vi "Init.vi"(0 "STOMP in":refnum<class "STOMP.lvclass">, 5 "error in (no error)":errorcluster) -> (14 "STOMP out":refnum<class "STOMP.lvclass">, 19 "error out":errorcluster)   [LabVIEW 2017, in "STOMP.lvclass"]
uses:
  STOMP.lvclass
  Typedefs/Type_ServerFrame.ctl
  Typedefs/Type_ServerFrameType.ctl
  Typedefs/ObjectAttributes.ctl
  Typedefs/Type_ActiveSubscription.ctl
  Typedefs/Type_AckHeader.ctl
  Typedefs/Type_FrameHeader.ctl
  STOMP.lvclass/STOMP.ctl
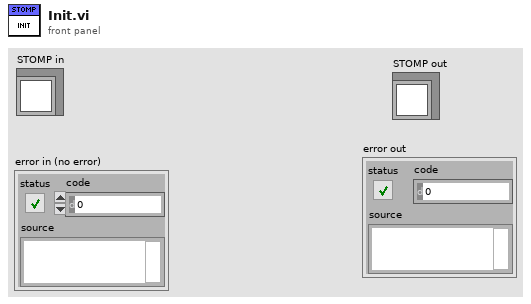
[diagram p1: front panel]
types:
  T1 = typedef "STOMP.lvclass/ObjectAttributes.ctl" = cluster{"address":string, "port":u16, "ConnectionRef":refnum<k5>, "messageQueue":refnum<queue>, "receiptQueue":refnum<queue>, "errorQueue":refnum<queue>, "sendQueue":refnum<queue>, "currentReceiptNumber":u64, "currentSubscriptionId":u64, "closeConnection":bool, "activeSubscriptions":T2[]}
  T2 = typedef "STOMP.lvclass/Type_ActiveSubscription.ctl" = cluster{"id":u64, "receipt":bool, "Destination":string, "ack":T3, "headers":T4[]}
  T3 = typedef "STOMP.lvclass/Type_AckHeader.ctl" = enum16{"auto", "client", "client-individual"}
  T4 = typedef "STOMP.lvclass/Type_FrameHeader.ctl" = cluster{"Header":string, "Value":string}
  T5 = typedef "STOMP.lvclass/Type_ServerFrame.ctl" = cluster{"Type":T6, "Headers":cluster{"Header":string, "Value":string}[], "Body":string}
  T6 = typedef "STOMP.lvclass/Type_ServerFrameType.ctl" = enum16{"Undefined", "MESSAGE", "CONNECTED", "RECEIPT", "ERROR"}
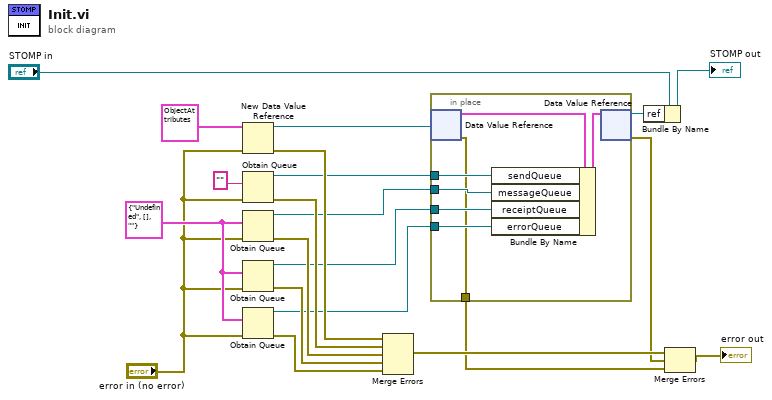
[diagram p0: block diagram]
diagram:
  w20 = T5 {"Type"=enum."Undefined", "Headers"=[], "Body"=""} ("Type_ServerFrame")
  n1 = New Data Value Reference(data value=T1 {"address"="", "port"=0, "ConnectionRef"=refnum, "messageQueue"=refnum, "receiptQueue"=refnum, "errorQueue"=refnum, "sendQueue"=refnum, "currentReceiptNumber"=0, "currentSubscriptionId"=0, "closeConnection"=FALSE, "activeSubscriptions"=[]} ("Cluster of class private data"), error in="error in (no error)") -> (data value reference=w12:refnum<data-value>, error out=w13:errorcluster)
  n2 = Obtain Queue(element data type="", error in (no error)="error in (no error)") -> (queue out=w11:refnum<queue>, error out=w16:errorcluster)  [unwired: 3 in, 1 out]
  n3 = Obtain Queue(element data type=w20, error in (no error)="error in (no error)") -> (queue out=w10:refnum<queue>, error out=w21:errorcluster)  [unwired: 3 in, 1 out]
  n4 = Obtain Queue(element data type=w20, error in (no error)="error in (no error)") -> (queue out=w9:refnum<queue>, error out=w19:errorcluster)  [unwired: 3 in, 1 out]
  n5 = Obtain Queue(element data type=w20, error in (no error)="error in (no error)") -> (queue out=w8:refnum<queue>, error out=w18:errorcluster)  [unwired: 3 in, 1 out]
  n6 = Merge Errors(w13, w16, w21, w19, w18) -> (w4:errorcluster)
  n7 = in-place {
    in-place-border: w11 -> [w27]
    in-place-border: w10 -> [w26]
    in-place-border: w9 -> [w25]
    in-place-border: w8 -> [w24]
    in-place-border: [w22] -> w2
    n8 = in-place-dvr #1(w12) -> (w28:T1, w22:errorcluster)
    n9 = Bundle By Name(cluster=w28, "sendQueue"=w27, "messageQueue"=w26, "receiptQueue"=w25, "errorQueue"=w24) -> (w23:T1)
    n10 = in-place-dvr #1(w23) -> (w5:refnum<data-value>, w3:errorcluster)
  }
  n11 = Bundle By Name(cluster="STOMP in", "ref"=w5) -> (→"STOMP out":refnum<class "STOMP.lvclass">)
  n12 = Merge Errors(w4, w3, w2) -> (→"error out":errorcluster)
